vi "SvgDoc Get H&W.vi"(8 "error in (no error)":errorcluster, 11 ".NET Refnum in":refnum<k24>) -> (0 "error out":errorcluster, 1 "Height":sgl, 2 "Width":sgl, 3 ".NET Refnum out":refnum<k24>)   [LabVIEW 2020, in "SvgDotNet.lvlib"]
uses:
  SvgDotNet.lvlib
  C:/Users/huipeng8/Desktop/SVG.NET/Svg.dll
  Svg.dll
panel:
  # "Connector Pane"
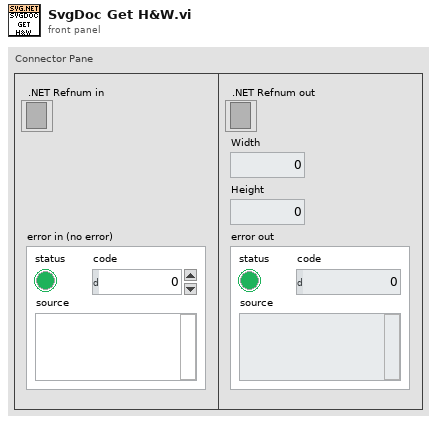
[diagram p1: front panel]
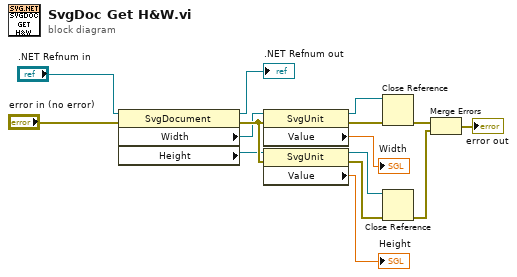
[diagram p0: block diagram]
diagram:
  n1 = property class="SvgDocument"(reference=".NET Refnum in", error in="error in (no error)") -> (reference out=→".NET Refnum out":refnum<k24>, error out=w5:errorcluster, "Width"=w3:refnum<k24>, "Height"=w4:refnum<k24>)
  n2 = property class="SvgUnit"(reference=w3, error in=w5) -> (reference out=w10:refnum<k24>, error out=w9:errorcluster, "Value"=→"Width":sgl)
  n3 = property class="SvgUnit"(reference=w4, error in=w5) -> (reference out=w11:refnum<k24>, error out=w12:errorcluster, "Value"=→"Height":sgl)
  n4 = Close Reference(reference=w10, error in (no error)=w9) -> (error out=w13:errorcluster)
  n5 = Close Reference(reference=w11, error in (no error)=w12) -> (error out=w14:errorcluster)
  n6 = Merge Errors(w13, w14) -> (→"error out":errorcluster)
